vi "Bounce.vi"(11 "Array":dbl[][](array[numeric])) -> (0 "Result calculated from":dbl[](array[numeric]), 1 "Acceleration":dbl, 2 "Time":dbl[](array[numeric]), 3 "Distance":dbl[](array[numeric]))   [LabVIEW 2021]
uses:
  <vilib>/Analysis/NI_AALPro.lvlib
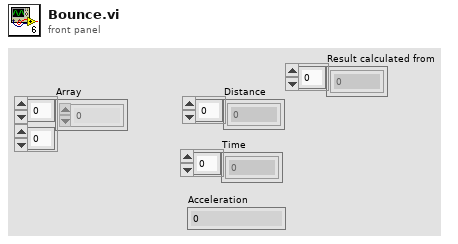
[diagram p1: front panel]
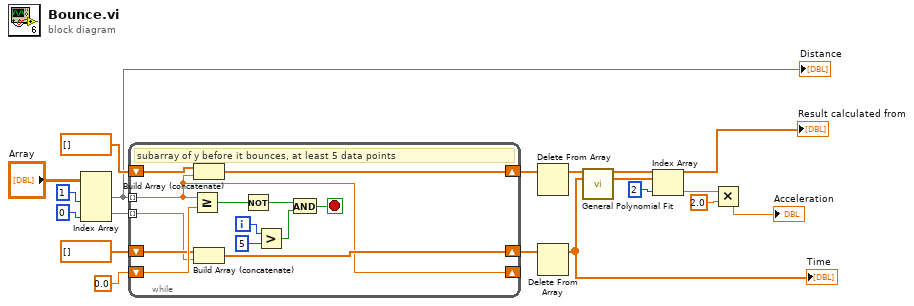
[diagram p0: block diagram]
diagram:
  n1 = Index Array(array="Array", index (col) #1=1 ("disabled index (col)"), index (col) #2=0 ("index (col)")) -> (element #1=w2:dbl[], element #2=w17:dbl[])  [unwired: 2 in]
  "Distance" <- w2
  n2 = while {
    tunnel: w2 -> [w18] mode=indexing
    tunnel: w17 -> [w19] mode=indexing
    shift-right: [w18] -> _
    shift-left: 0.0 -> [w30]
    shift-right: [w26] -> w15
    shift-left: dbl[] [] -> [w27]
    shift-right: [w25] -> w16
    shift-left: dbl[] [] -> [w28]
    i -> [w24]
    stop <- w20 stop-if-true
    # "subarray of y before it bounces, at least 5 data points"
    n3 = Greater Or Equal?(x=w18, y=w30) -> (x >= y?=w29:bool)
    n4 = Build Array (concatenate)(w27, w18) -> (w26:dbl[])
    n5 = Build Array (concatenate)(w28, w19) -> (w25:dbl[])
    n6 = Not(x=w29) -> (.not. x?=w21:bool)
    n7 = Greater?(x=w24, y=5) -> (0:w22:bool)
    n8 = And(x=w21, y=w22) -> (x .and. y?=w20:bool)
  }
  n9 = Delete From Array(array=w15) -> (array with subset deleted=w1:dbl[])  [unwired: 2 in, 1 out]
  "Result calculated from" <- w1
  n10 = Delete From Array(array=w16) -> (array with subset deleted=w3:dbl[])  [unwired: 2 in, 1 out]
  "Time" <- w3
  n11 = call <vilib>:"General Polynomial Fit.vi"("Y"=w1, "X"=w3) -> ("Polynomial Coefficients"=w7:dbl[])  [unwired: 10 in, 3 out]
  n12 = Index Array(array=w7, index=2) -> (element=w8:dbl)
  n13 = Multiply(x=w8, y=2.0) -> (x*y=→"Acceleration":dbl)
